vi "Flatten Value.vi"(8 "error in":errorcluster, 11 "2D Path In":refnum<class "2D Path.lvclass">) -> (0 "error out":errorcluster, 1 "Value":string, 3 "2D Path Out":refnum<class "2D Path.lvclass">)   [LabVIEW 2020, in "NI_VIAnCFGDataStructure.lvlib" / "2D Path.lvclass"]
doc: "Dynamic dispatch interface for flattening Tree Data classes to string."
uses:
  <vilib>/addons/analyzer/VIAnCFGDataStructure/Data Types/2D Path/2D Path.lvclass
  <vilib>/addons/analyzer/VIAnCFGDataStructure/Data Types/2D Path/2D Path.lvclass/2D Path.ctl
  <vilib>/addons/analyzer/VIAnCFGDataStructure/Tree Manager/API/Generate Hash.vi
  <vilib>/addons/analyzer/VIAnCFGDataStructure/Tree Manager/Tree.lvclass
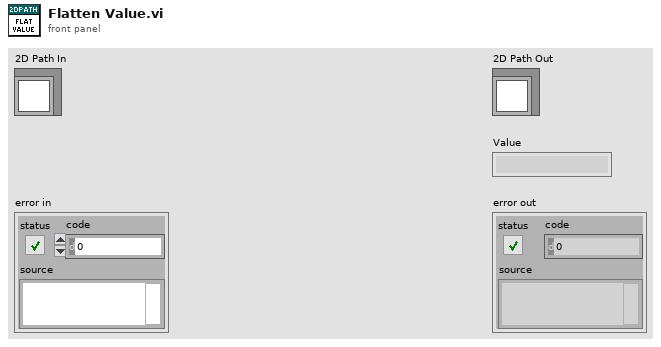
[diagram p1: front panel]
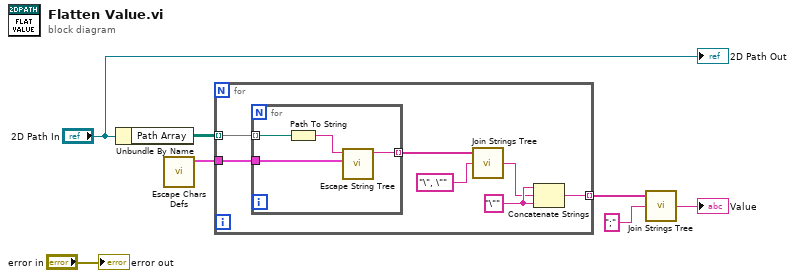
[diagram p0: block diagram]
diagram:
  n1 = Unbundle By Name("2D Path In") -> ("Path Array"=w7:path[][])
  n2 = call <vilib>:"Escape Chars Defs.vi"() -> ("Escapes"=w1:cluster{"String":string, "Escape":string}[])  [unwired: 11 in]
  n3 = for {
    tunnel: w7 -> [w14] mode=indexing
    tunnel: [w9] -> w5 mode=indexing
    tunnel: w1 -> [w8]
    w12 = "\"" ("string")
    n4 = for {
      tunnel: w14 -> [w18] mode=indexing
      tunnel: [w16] -> w10 mode=indexing
      tunnel: w8 -> [w15]
      n5 = Path To String(path=w18) -> (string=w17:string)
      n6 = call <vilib>:"Escape String Tree.vi"("Escapes"=w15, "String In"=w17) -> ("String Out"=w16:string)  [unwired: 9 in]
    }
    n7 = call <vilib>:"Join Strings Tree.vi"("Separator (,)"="\", \"", "Strings In"=w10) -> ("String"=w11:string)  [unwired: 1 in]
    n8 = Concatenate Strings(w12, w11, w12) -> (w9:string)
  }
  n9 = call <vilib>:"Join Strings Tree.vi"("Separator (,)"=";", "Strings In"=w5) -> ("String"=→"Value":string)  [unwired: 1 in]
  "2D Path Out" <- "2D Path In"
  "error out" <- "error in"
